vi "Open TCP.vi"(4 "Timeout":i32, 8 "error in (no error)":errorcluster, 9 "Port":u16, 10 "Network Address":string) -> (0 "error out":errorcluster, 2 "Device Name":string, 3 "LINX Client out":refnum<class "LINX Client.lvclass">)   [LabVIEW 2020, in "LINX Client.lvclass"]
uses:
  LINX Client.lvclass
  LINX Client.lvclass/LINX Client.ctl
  LINX Base.lvclass
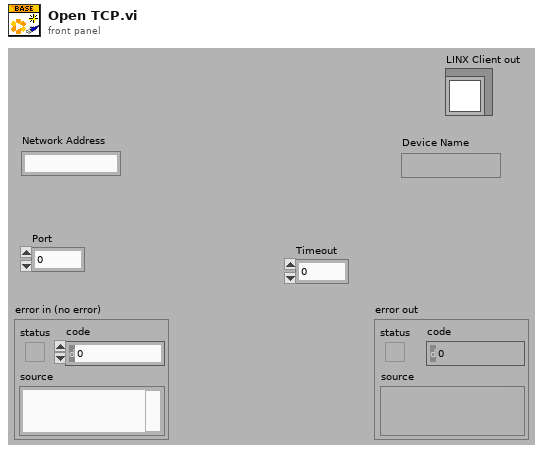
[diagram p1: front panel]
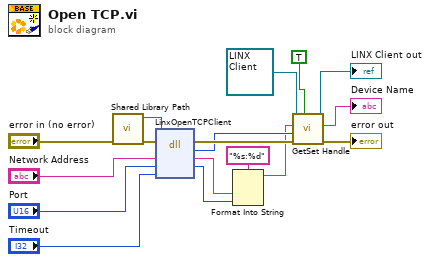
[diagram p0: block diagram]
diagram:
  n1 = call "Shared Library Path.vi"("error in (no error)"="error in (no error)") -> ("error out"=w17:errorcluster, "Path"=w16:path)  [unwired: 9 out]
  n2 = dll-call lib="Z:/Development/LabVIEW Hobbyist Toolkit/LabVIEW/vi.lib/MakerHub/LINX/Resources/libLinxDevice.dll" fn="LinxOpenTCPClient"(path in=w16, error in=w17, "address"="Network Address", "port"="Port", "timeout"="Timeout") -> (error out=w11:errorcluster, "LinxDevice"=w10:u64, "address"=w9:string, "port"=w8:u16)  [unwired: 2 in, 1 out]
  n3 = Format Into String(format string="%s:%d", w9, w8) -> (resulting string=w2:string)  [unwired: 2 in, 1 out]
  n4 = call-dynamic "GetSet Handle.vi"("store (F)"=TRUE, "error in"=w11, "handle in"=w10, "connection"=w2, "LINX Base in"=refnum<class "LINX Client.lvclass"> refnum ("LINX Device")) -> ("error out"=→"error out":errorcluster, "name"=→"Device Name":string, "LINX Base out"=→"LINX Client out":refnum<class "LINX Client.lvclass">)  [unwired: 1 in, 3 out]
